vi "MCListbox Event - Mouse Down.vi"(8 "Error In":errorcluster, 11 "CtlRef":refnum<vi>) -> (0 "Error Out":errorcluster)   [LabVIEW 2013]
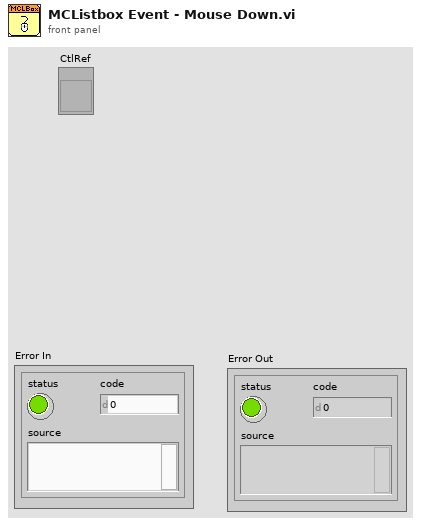
[diagram p1: front panel]
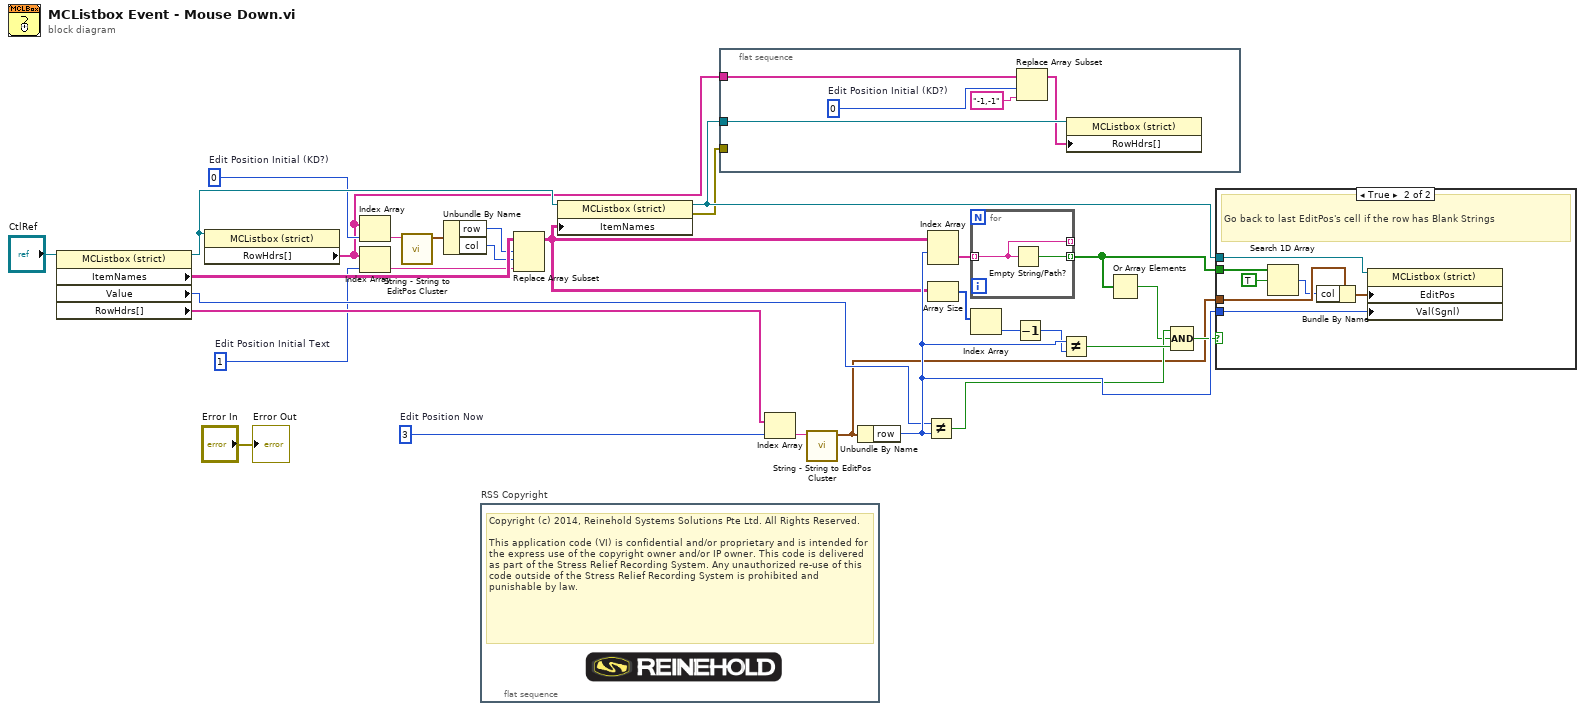
[diagram p0: block diagram]
diagram:
  w5 = 1  # Edit Position Initial Text
  w6 = 0  # Edit Position Initial (KD?)
  w12 = 3  # Edit Position Now
  n1 = property on="Property Node" class="MCListbox (strict)"(reference="CtlRef") -> (reference out=w20:refnum<vi>, "ItemNames"=w19:string[][], "Value"=w25:i32, "RowHdrs[]"=w13:string[])  [unwired: 1 in, 1 out]
  n2 = property on="Property Node" class="MCListbox (strict)"(reference=w20) -> ("RowHdrs[]"=w3:string[])  [unwired: 1 in, 2 out]
  n3 = Index Array(array=w3, index=w6) -> (element=w2:string)
  n4 = Index Array(array=w3, index=w5) -> (element=w4:string)
  n5 = call "String - String to EditPos Cluster.vi"("string"=w2) -> ("EditPos"=w1:cluster{"row":i32, "col":i32})  [unwired: 10 in]
  n6 = Unbundle By Name(w1) -> ("row"=w9:i32, "col"=w8:i32)
  n7 = flat-sequence "RSS Copyright" {
    frame #0 {
      # "Copyright (c) 2014, Reinehold Systems Solutions Pte Ltd. All Rights Reserved.\n\nThis application code (VI) is confidential and/or proprietary and is intended for the express use of the copyright owner and/or IP owner. This code is delivered as part of the Stress Relief Recording System. Any unauthorized re-use of this code outside of the Stress Relief Recording System is prohibited and punishable by law."
    }
  }
  n8 = Replace Array Subset(array=w19, new element=w4, index (row)=w9, index (col)=w8) -> (w23:string[][])
  n9 = property on="Property Node" class="MCListbox (strict)"(reference=w20, "ItemNames"=w23) -> (reference out=w21:refnum<vi>, error out=w7:errorcluster)  [unwired: 1 in]
  n10 = flat-sequence {
    tunnel: w7 -> [_]
    tunnel: w21 -> [w35]
    tunnel: w3 -> [w34]
    frame #0 {
      w33 = 0  # Edit Position Initial (KD?)
      n11 = Replace Array Subset(array=w34, new element="-1,-1" ("new element/subarray"), index=w33) -> (w31:string[])
      n12 = property on="Property Node" class="MCListbox (strict)"(reference=w35, "RowHdrs[]"=w31) -> ()  [unwired: 1 in, 2 out]
    }
  }
  n13 = Index Array(array=w13, index=w12) -> (element=w11:string)
  n14 = call "String - String to EditPos Cluster.vi"("string"=w11) -> ("EditPos"=w10:cluster{"row":i32, "col":i32})  [unwired: 10 in]
  n15 = Unbundle By Name(w10) -> ("row"=w28:i32)
  n16 = Not Equal?(x=w25, y=w28) -> (x != y?=w17:bool)
  n17 = Index Array(array=w23, index (row)=w28) -> (element=w15:string[])  [unwired: 1 in]
  n18 = Array Size(array=w23) -> (size(s)=w24:i32[])
  n19 = for {
    tunnel: [w37] -> _ mode=indexing
    tunnel: w15 -> [w37] mode=indexing
    tunnel: [w36] -> w22 mode=indexing
    n20 = Empty String/Path?(string/path=w37) -> (empty?=w36:bool)
  }
  n21 = Index Array(array=w24) -> (element=w26:i32)  [unwired: 1 in]
  n22 = Decrement(x=w26) -> (x-1=w27:i32)
  n23 = Not Equal?(x=w28, y=w27) -> (x != y?=w29:bool)
  n24 = Or Array Elements(Boolean array=w22) -> (logical OR=w16:bool)
  n25 = Compound Arithmetic op=AND(w17, w16, w29) -> (w18:bool)
  n26 = case shown="True" w18 {
    tunnel: w10 -> [_ w40]
    tunnel: w28 -> [_ w43]
    tunnel: w21 -> [_ w44]
    tunnel: w22 -> [_ w42]
    frame False {
    }
    frame True {
      # "Go back to last EditPos's cell if the row has Blank Strings"
      n27 = Search 1D Array(1D array=w42, element=TRUE) -> (index of element=w39:i32)  [unwired: 1 in]
      n28 = Bundle By Name(cluster=w40, "col"=w39) -> (w38:cluster{"row":i32, "col":i32})
      n29 = property on="Property Node" class="MCListbox (strict)"(reference=w44, "EditPos"=w38, "Val(Sgnl)"=w43) -> ()  [unwired: 1 in, 2 out]
    }
  }
  "Error Out" <- "Error In"
